vi "Prueba filtros.vi"() -> ()   [LabVIEW 2023]
uses:
  <vilib>/Analysis/3filter.llb/Filter Passband Type.ctl
  <vilib>/express/express analysis/Spectral/Block/exnSpectralBlock spectral measurements power poly.vi
  <vilib>/express/express analysis/Spectral/Block/exnSpectralBlock spectral measurements power DDT.vi
  <vilib>/Waveform/WDTOps.llb/WDT Get Waveform Time Array DBL.vi
  <vilib>/Analysis/3filter.llb/Butterworth Filter (DBL).vi
  <vilib>/express/express analysis/Spectral/XNode/ExpressSpectralMeasurementsBlockNode.xnode
  <vilib>/Analysis/NI_AALBase.lvlib
panel:
  in  "Reproducir sonido Filtrado":bool
  in  "Stop":bool
  out "Espectro Waveform":dynamicdata(graph)
  in  "Actualizar Filtro":bool
  in  "Tipo de Filtro":T1
  in  "Orden":i32=2
  in  "Frecuencia de corte baja":dbl=0.12500000000000006 format="%0.4f"
  in  "Frecuencia de corte alta":dbl=0.45000000000000007 format="%0.2f"
  out "Señal Obtenida":dynamicdata(graph) caption="Data"
  in  "Tiempo de la Grabacion (s)":dbl=1.0 caption="Duration (s)"
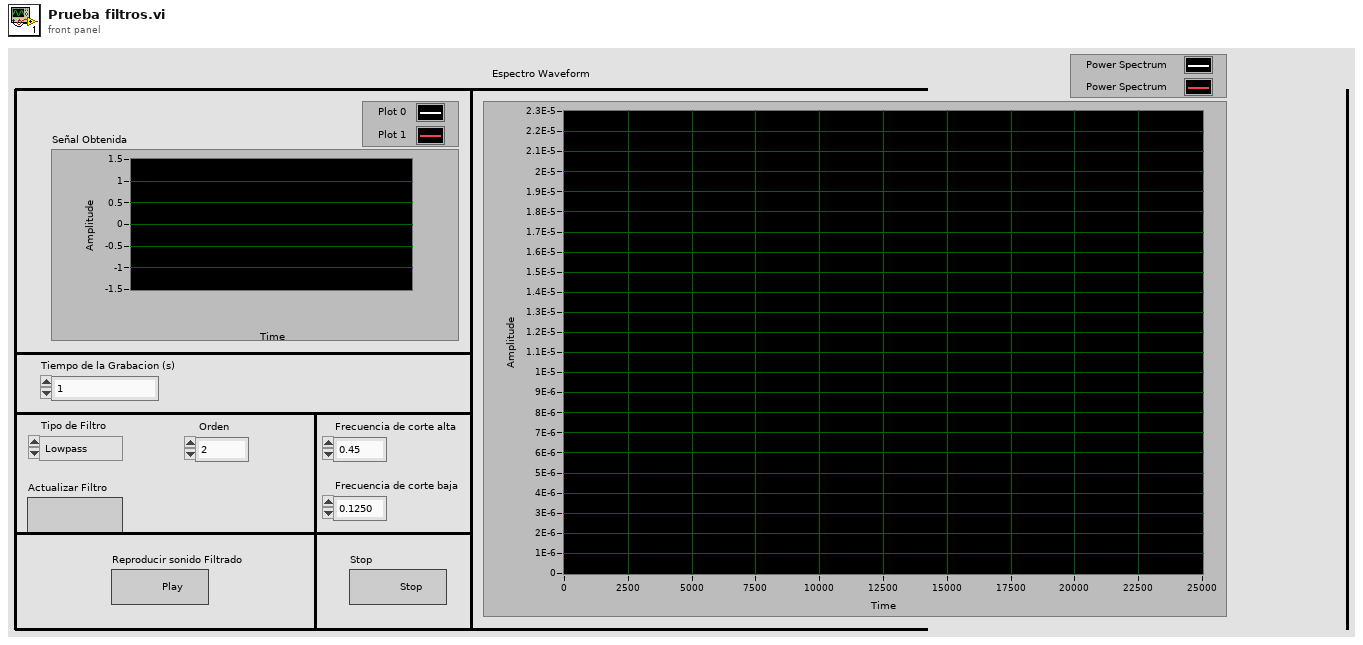
[diagram p1: front panel]
types:
  T1 = typedef "NI_AALBase.lvlib/Filter Passband Type.ctl" = enum32{"Lowpass", "Highpass", "Bandpass", "Bandstop"}
  T2 = cluster{"averaging mode":u16, "weighting mode":u16, "number of averages":u32}
  T3 = cluster{"dB On (F)":bool, "unwrap phase (F)":bool, "convert to degree (F)":bool}
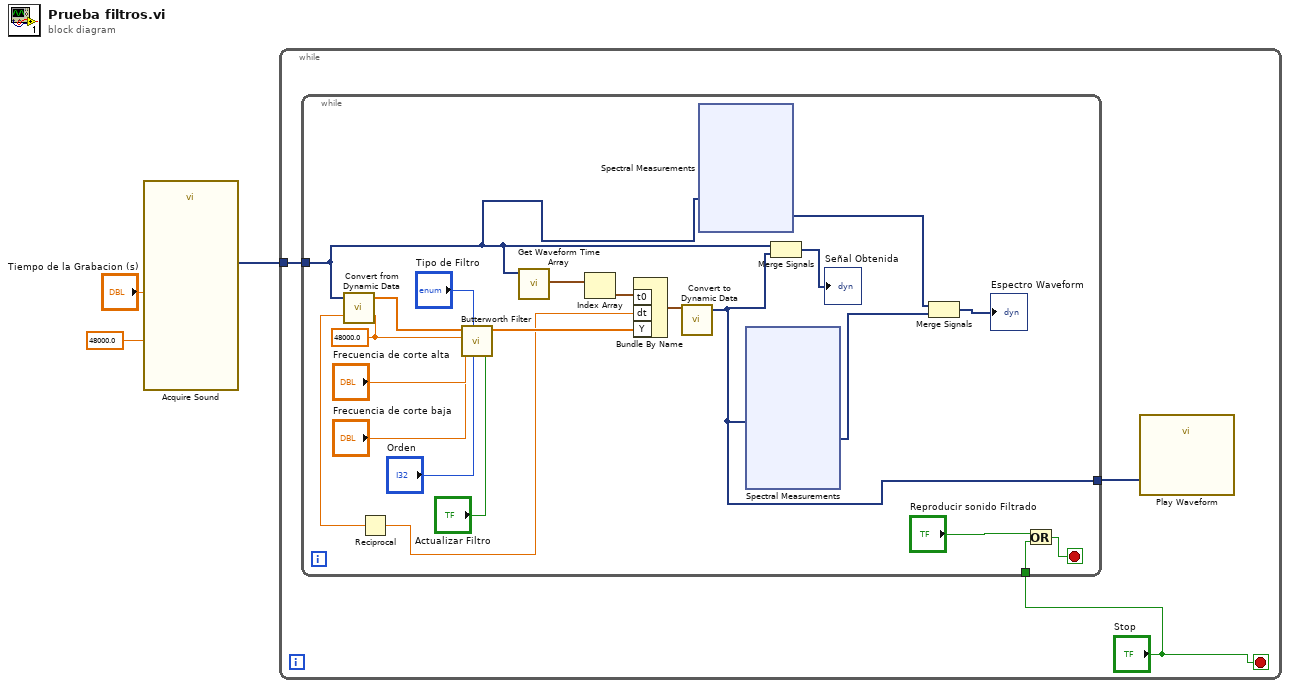
[diagram p0: block diagram]
diagram:
  n1 = call "Acquire Sound"("Duration (s)"="Tiempo de la Grabacion (s)", "Sample rate (Hz)"=48000.0) -> ("Data"=w1:dynamicdata)  [unwired: 16 in, 1 out]
  n2 = while {
    tunnel: w1 -> [w4]
    stop <- "Stop" stop-if-true
    n3 = while {
      tunnel: [w9] -> w6
      tunnel: "Stop" -> [w18]
      tunnel: w4 -> [w8]
      stop <- w16 stop-if-true
      w15 = 48000.0 ("sampling freq: fs")
      n4 = call "Convert from Dynamic Data"("Dynamic Data Type"=w8) -> ("Array"=w27:dbl[])  [unwired: 3 in]
      n5 = Reciprocal(x=w15) -> (1/x=w11:dbl)
      n6 = call-poly <vilib>:"Butterworth Filter.vi"("init/cont (init:F)"="Actualizar Filtro", "order"="Orden", "filter type"="Tipo de Filtro", "low cutoff freq: fl"="Frecuencia de corte baja", "high cutoff freq: fh"="Frecuencia de corte alta", "sampling freq: fs"=w15, "X"=w27) -> ("Filtered X"=w14:dbl[])  [unwired: 1 in, 1 out]
      n7 = call-poly <vilib>:"Get Waveform Time Array.vi"("waveform in"=w8) -> ("X array"=w13:timestamp[])  [unwired: 9 in, 1 out]
      n8 = Index Array(array=w13) -> (element=w12:timestamp)  [unwired: 1 in]
      n9 = Bundle By Name("t0"=w12, "dt"=w11, "Y"=w14) -> (w10:waveform(dbl))  [unwired: 1 in]
      n10 = call "Convert to Dynamic Data"("Waveform"=w10) -> ("Dynamic Data Type"=w9:dynamicdata)  [unwired: 3 in]
      n11 = xnode "Spectral Measurements"("Signals"=w8) -> ("Power Spectrum"=w7:dynamicdata)  [unwired: 1 in, 1 out]
      n12 = xnode "Spectral Measurements"("Signals"=w9) -> ("Power Spectrum"=w20:dynamicdata)  [unwired: 1 in, 1 out]
      n13 = Merge Signals(w8, w9) -> (→"Señal Obtenida":dynamicdata)
      n14 = Merge Signals(w7, w20) -> (→"Espectro Waveform":dynamicdata)
      n15 = Or(x="Reproducir sonido Filtrado", y=w18) -> (x .or. y?=w16:bool)
    }
    n16 = call "Play Waveform"("Data"=w6) -> ()  [unwired: 18 in, 1 out]
  }
